vi "readFreqData.vi"(0 "FrequencyCounter.lvclass":refnum<class "FrequencyCounter.lvclass">, 1 "error in (no error)":errorcluster) -> (2 "FrequencyCounter.lvclass 2":refnum<class "FrequencyCounter.lvclass">, 3 "String":string, 4 "error out":errorcluster)   [LabVIEW 2011, in "Hardware.lvlib" / "frequencyCounters.lvlib" / "FrequencyCounter.lvclass"]
uses:
  FrequencyCounter.lvclass
  FrequencyCounter.lvclass/FrequencyCounter.ctl
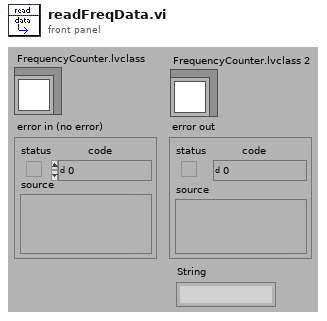
[diagram p1: front panel]
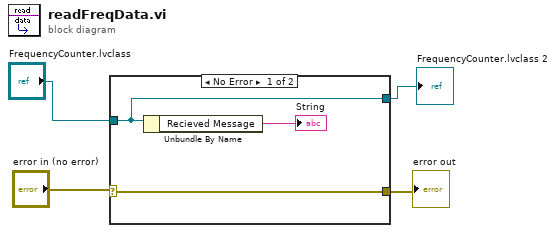
[diagram p0: block diagram]
diagram:
  n1 = case shown="No Error" "error in (no error)" {
    selector: "error in (no error)" -> [w5 w8]
    tunnel: "FrequencyCounter.lvclass" -> [w6 w9]
    tunnel: [w6 w9] -> w2
    tunnel: [w5 w8] -> w1
    frame No Error {
      n2 = Unbundle By Name(w6) -> ("Recieved Message"=→"String":string)
    }
    frame Error {
    }
  }
  "error out" <- w1
  "FrequencyCounter.lvclass 2" <- w2
